vi "create_attribute_error.vi"(4 "Original error splitter\n(\"Original error:\")":string="\nOriginal error:\n", 5 "Error Elaboration (\"\")":string, 6 "Error creation enabled (T)":bool=TRUE, 7 "Attribute":T2={"Identifier"="", "Descriptive name"="", "Data Type"=enum."Integer 32", "Command"="", "Access"=2, "Range Table"="", "Read Callback"="", "Write Callback"="", "Range Callback"="", "Check Callback"="", "Rngtable Callback"="", "Coerce Callback"="", "Supported Models"="", "Instrument Options"="", "Repeated Capabilities"="", "Check Status Callback"="", "Index"=0, "Flag: OPC Wait"=FALSE, "Flag: Dont check status"=FALSE, "Flag: Cache Only"=FALSE} {"Access" items=["Read Only", "Write Only", "Read/Write"]}, 8 "error in":errorcluster, 9 "Additional detail from error source (\"\")":string, 10 "Error Enum in":T1=enum."VISA_err_Timeout", 11 "VISA resource name":refnum<visa-resource-name>) -> (0 "error out":errorcluster, 3 "VISA resource name out":refnum<visa-resource-name>)   [LabVIEW 2014, in "rszvl_rsidr_core.lvlib"]
uses:
  rszvl_rsidr_core.lvlib
  type_Attribute.ctl
  type_Attribute_Data_Type.ctl
  type_Error_Codes.ctl
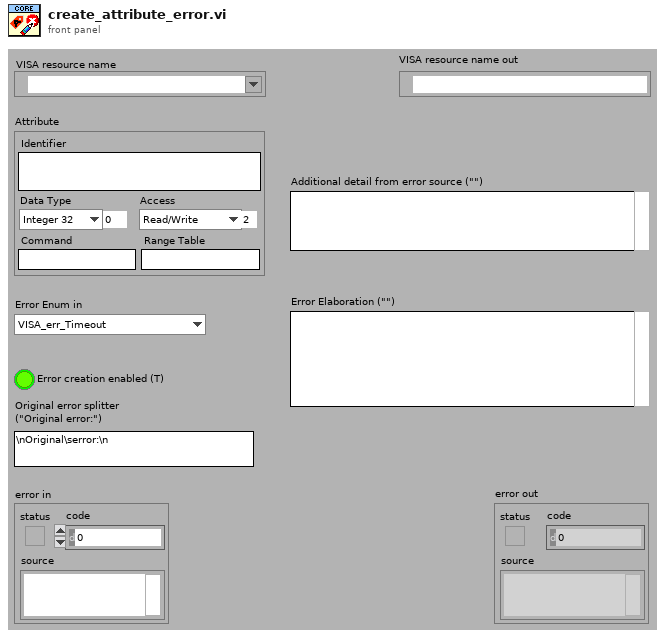
[diagram p1: front panel]
types:
  T1 = typedef "rszvl_rsidr_core.lvlib/type_Error_Codes.ctl" = enum16{"No_error", "VISA_err_ResourceNotFound", "VISA_err_Timeout", "VISA_warn_MoreDataAvailable", "RS_err_MissingCallback", "RS_err_InvalidAttribute", "RS_err_InvalidValue", "RS_err_UnknownResource", "RS_err_AlreadyInitialized", "RS_err_InstrumentStatus", "RS_err_BadRepCapName", "RS_err_TypesMismatch", "RS_err_ValueNotSupported", "RS_err_InvalidRngTable", "RS_err_IDqueryFail", "RS_err_UnexpResponse", "VISA_warn_ConfigNotLoaded", "RS_err_AttributeNotReadable", "RS_err_AttributeNotWritable", "RS_err_InstrumentType", "RS_err_InstrumentOption", "VISA_err_InvalidSize", "RS_err_ReliabilityIndicator", "VISA_warn_UnknownStatus", "VISA_warn_TermCharRead", "VISA_err_IO_error"}
  T2 = typedef "rszvl_rsidr_core.lvlib/type_Attribute.ctl" = cluster{"Identifier":string, "Descriptive name":string, "Data Type":T3, "Command":string, "Access":u16, "Range Table":string, "Read Callback":string, "Write Callback":string, "Range Callback":string, "Check Callback":string, "Rngtable Callback":string, "Coerce Callback":string, "Supported Models":string, "Instrument Options":string, "Repeated Capabilities":string, "Check Status Callback":string, "Index":i32, "Flag: OPC Wait":bool, "Flag: Dont check status":bool, "Flag: Cache Only":bool}
  T3 = typedef "rszvl_rsidr_core.lvlib/type_Attribute_Data_Type.ctl" = enum16{"Integer 32", "Double", "String", "Boolean", "None", "Integer 64"}
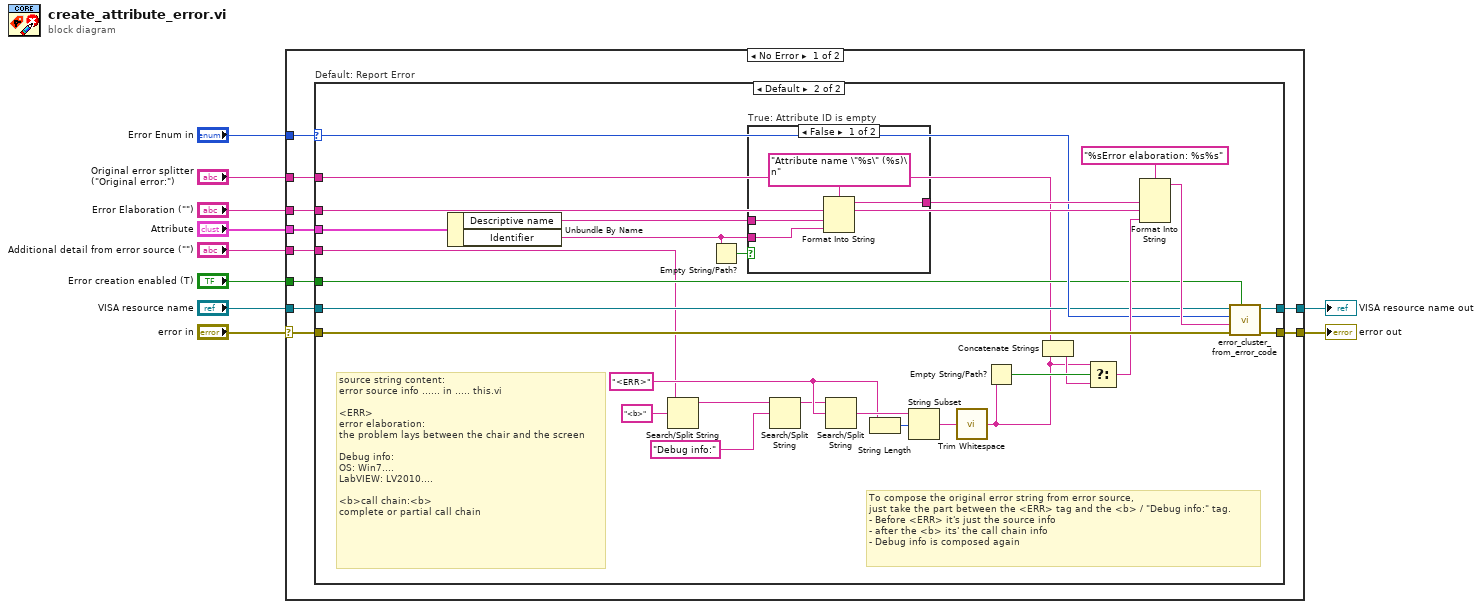
[diagram p0: block diagram]
diagram:
  n1 = case shown="No Error" "error in" {
    selector: "error in" -> [w17 w56]
    tunnel: "Attribute" -> [w18 _]
    tunnel: "Error Elaboration (\"\")" -> [w19 _]
    tunnel: [w20 w56] -> w9
    tunnel: "Error Enum in" -> [w16 _]
    tunnel: "VISA resource name" -> [w15 w55]
    tunnel: [w14 w55] -> w4
    tunnel: "Original error splitter\n(\"Original error:\")" -> [w13 _]
    tunnel: "Error creation enabled (T)" -> [w12 _]
    tunnel: "Additional detail from error source (\"\")" -> [w11 _]
    frame No Error {
      n2 = case "Default: Report Error" shown="Default" w16 {
        selector: w16 -> [_ w31]
        tunnel: [w22 w47] -> w20
        tunnel: w17 -> [w22 w48]
        tunnel: w18 -> [_ w50]
        tunnel: w19 -> [_ w49]
        tunnel: w15 -> [w21 w30]
        tunnel: [w21 w29] -> w14
        tunnel: w13 -> [_ w23]
        tunnel: w12 -> [_ w25]
        tunnel: w11 -> [_ w24]
        frame "No_error" {
        }
        frame Default {
          w38 = "<ERR>" ("search string/char (-)")
          # "source string content:\nerror source info ...... in ..... this.vi\n\n<ERR>\nerror elaboration:\nthe problem lays between the chair and the screen\n\nDebug info:\nOS: Win7....\nLabVIEW: LV2010....\n\n<b>call chain:<b>\ncomplete or partial call chain"
          # "To compose the original error string from error source,\njust take the part between the <ERR> tag and the <b> / \"Debug info:\" tag.\n- Before <ERR> it's just the source info\n- after the <b> its' the call chain info\n- Debug info is composed again"
          n3 = Unbundle By Name(w50) -> ("Descriptive name"=w42:string, "Identifier"=w44:string)
          n4 = Search/Split String(string=w24, search string/char (-)="<b>") -> (substring before match=w28:string)  [unwired: 1 in, 2 out]
          n5 = Empty String/Path?(string/path=w44) -> (empty?=w45:bool)
          n6 = case "True: Attribute ID is empty" shown="False" w45 {
            tunnel: w44 -> [w51 _]
            tunnel: [w53 _] -> w43
            tunnel: w42 -> [w52 _]
            frame False {
              n7 = Format Into String(format string="Attribute name \"%s\" (%s)\n", w52, w51) -> (resulting string=w53:string)  [unwired: 2 in, 1 out]
            }
            frame True {
            }
          }
          n8 = Search/Split String(string=w28, search string/char (-)="Debug info:") -> (substring before match=w26:string)  [unwired: 1 in, 2 out]
          n9 = Search/Split String(string=w26, search string/char (-)=w38) -> (match + rest of string=w40:string)  [unwired: 1 in, 2 out]
          n10 = String Length(string=w38) -> (length=w39:i32)
          n11 = String Subset(string=w40, offset (0)=w39) -> (substring=w37:string)  [unwired: 1 in]
          n12 = call "Trim Whitespace.vi"("string"=w37) -> ("trimmed string"=w33:string)  [unwired: 1 in]
          n13 = Empty String/Path?(string/path=w33) -> (empty?=w36:bool)
          n14 = Concatenate Strings(w23, w33) -> (w34:string)
          n15 = Select(t=w33, s=w36, f=w34) -> (s? t:f=w35:string)
          n16 = Format Into String(format string="%sError elaboration: %s%s", w43, w49, w35) -> (resulting string=w32:string)  [unwired: 2 in, 1 out]
          n17 = call "error_cluster_from_error_code.vi"("error creation enabled (T)"=w25, "error in"=w48, "error message (\"\")"=w32, "Error Enum in"=w31, "VISA resource name"=w30) -> ("error out"=w47:errorcluster, "VISA resource name out"=w29:refnum<visa-resource-name>)  [unwired: 5 in]
        }
      }
    }
    frame Error {
    }
  }
  "error out" <- w9
  "VISA resource name out" <- w4
